vi "Build Application with API.vi"(8 "error in (no error)":errorcluster, 11 "PostBuildSupport in":refnum<class "PostBuildSupport.lvclass">) -> (0 "error out":errorcluster, 3 "PostBuildSupport out":refnum<class "PostBuildSupport.lvclass">)   [LabVIEW 2016, in "PostBuildSupport.lvclass"]
uses:
  PostBuildSupport.lvclass
  PostBuildSupport.lvclass/PostBuildSupport.ctl
  <vilib>/AppBuilder/AB_API/EXE/NI_AB_API_EXE.lvclass
panel:
  in  "Cancel Button":bool
  out "Progress Bar":u8(slide) caption="The build is complete. You can locate the build at\nC:\\user\\patrick\\git\\PPMS-Monitor-and-Control\\builds\\PPMS Monitor and Control\\Application." scale=0.0..100.0
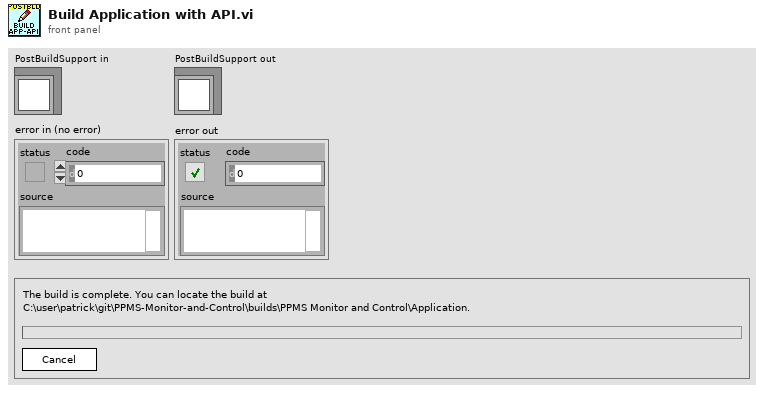
[diagram p1: front panel]
types:
  T1 = enum8{"Enabled", "Disabled", "Disabled and Grayed Out"}
  T2 = typedef "AB_API ProgressBar_Events.ctl" = cluster{"newJob":refnum<user-event>, "newItem":refnum<user-event>, "errorMsg":T3, "cancel":refnum<user-event>}
  T3 = typedef "AB_API ProgressBar_BuildError.ctl" = refnum<user-event>
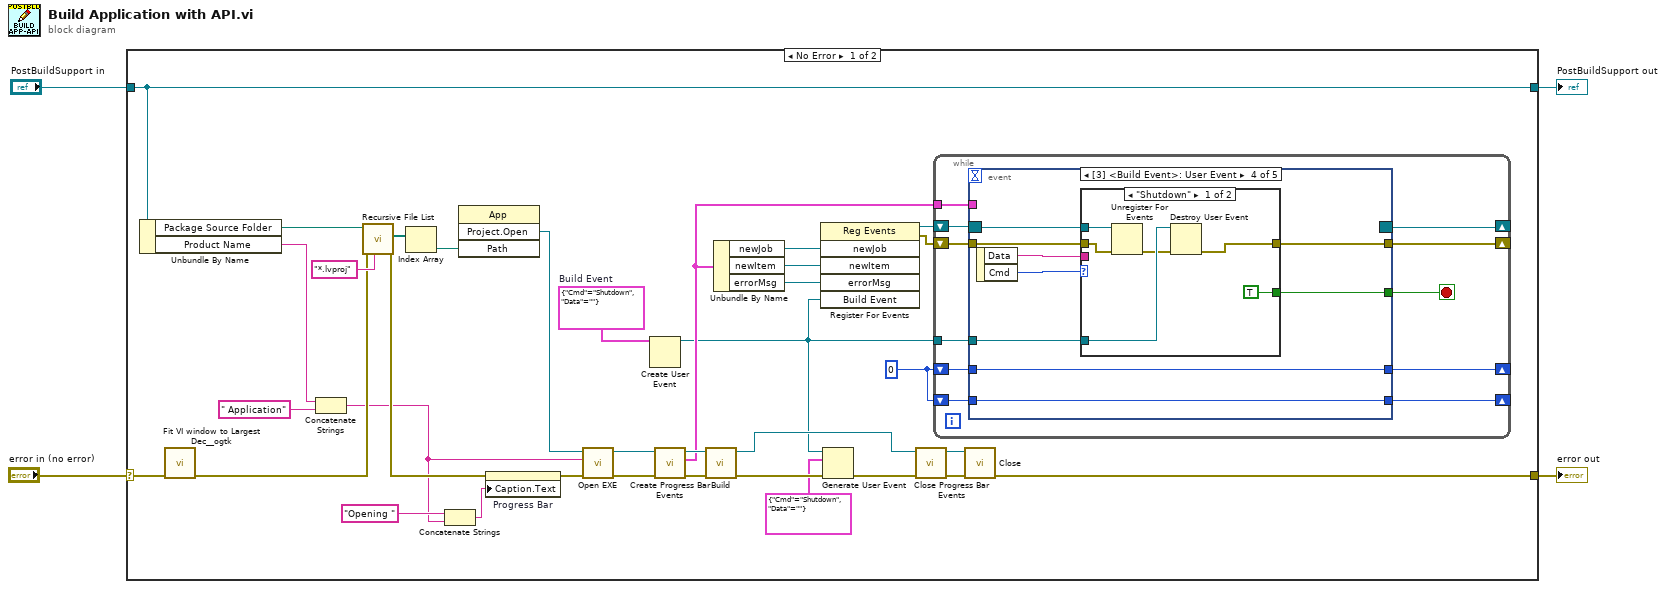
[diagram p0: block diagram]
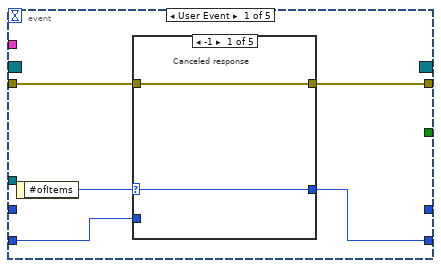
[diagram p2: hidden frame]
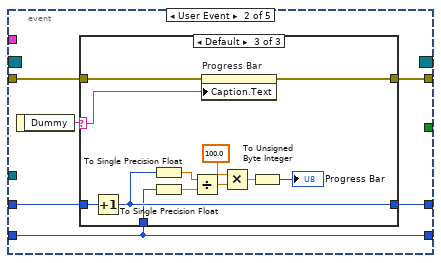
[diagram p7: hidden frame]
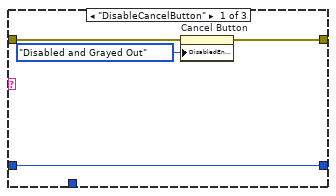
[diagram p8: hidden frame]
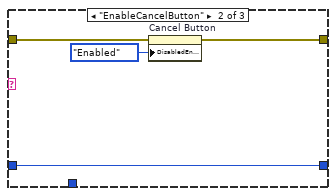
[diagram p9: hidden frame]
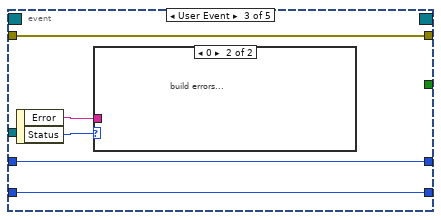
[diagram p10: hidden frame]
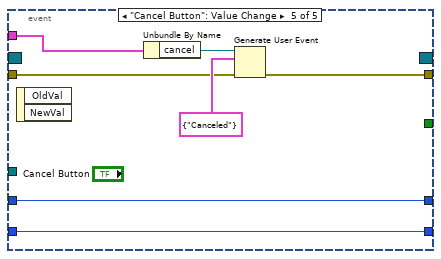
[diagram p13: hidden frame]
diagram:
  n1 = case shown="No Error" "error in (no error)" {
    selector: "error in (no error)" -> [w30 w121]
    tunnel: "PostBuildSupport in" -> [w38 w120]
    tunnel: [w36 w121] -> w2
    tunnel: [w38 w120] -> w1
    frame No Error {
      w19 = cluster{"Cmd":enum16{"Shutdown"}, "Data":string} {"Cmd"=enum."Shutdown", "Data"=""}  # Build Event
      w18 = 0 ("#ofItems")
      n2 = Unbundle By Name(w38) -> ("Package Source Folder"=w32:path, "Product Name"=w33:string)
      n3 = call <userlib>:"Fit VI window to Largest Dec__ogtk.vi"("error in (no error)"=w30) -> ("error out"=w7:errorcluster)  [unwired: 5 in, 1 out]
      n4 = Concatenate Strings(w33, " Application" ("Name of target (My Computer)")) -> (w5:string)
      n5 = call <vilib>:"Recursive File List.vi"("pattern"="*.lvproj", "error in (no error)"=w7, "Folder Path"=w32) -> ("error out"=w6:errorcluster, "All Files in Dir"=w39:path[])  [unwired: 4 in, 3 out]
      n6 = Index Array(array=w39) -> (element=w35:path)  [unwired: 1 in]
      n7 = Concatenate Strings("Opening " ("string"), w5) -> (w9:string)
      n8 = invoke class="App" method="Project.Open"("Path"=w35) -> ("Project:Open"=w34:refnum<vi>)  [unwired: 3 in, 3 out]
      n9 = property on="Progress Bar" class="Slide (strict)"(error in=w6, "Caption.Text"=w9) -> (error out=w10:errorcluster)  [unwired: 1 in, 1 out]
      n10 = call <vilib>:"Open EXE.vi"("error in (no error)"=w10, "Build specification name"=w5, "Project Refnum"=w34) -> ("error out"=w11:errorcluster, "EXE out"=w12:refnum<class "NI_AB_API_EXE.lvclass">)  [unwired: 7 in]
      n11 = Create User Event(user event datatype=w19) -> (user event=w14:refnum<user-event>)  [unwired: 1 in, 1 out]
      n12 = call-dynamic "Create Progress Bar Events.vi"("error in (no error)"=w11, "NI_AB_API_Build in"=w12) -> ("error out"=w25:errorcluster, "progressBarEvents"=w17:T2, "NI_AB_API_Build out"=w29:refnum<class "NI_AB_API_EXE.lvclass">)  [unwired: 7 in]
      n13 = call-dynamic "Build.vi"("error in (no error)"=w25, "EXE in"=w29) -> ("error out"=w16:errorcluster, "EXE out"=w28:refnum<class "NI_AB_API_EXE.lvclass">)  [unwired: 6 in, 2 out]
      n14 = Unbundle By Name(w17) -> ("newJob"=w24:refnum<user-event>, "newItem"=w23:refnum<user-event>, "errorMsg"=w22:T3)
      n15 = register-events(w24, w23, w22, w14) -> (reference out=w21:refnum<event-registration>, error out=w20:errorcluster)  [unwired: 2 in]
      n16 = Generate User Event(user event=w14, event data cluster=cluster{"Cmd":enum16{"Shutdown"}, "Data":string} {"Cmd"=enum."Shutdown", "Data"=""} ("event data"), error in=w16) -> (error out=w15:errorcluster)  [unwired: 1 in, 1 out]
      n17 = call-dynamic "Close Progress Bar Events.vi"("error in (no error)"=w15, "NI_AB_API_Build in"=w28) -> ("error out"=w26:errorcluster, "NI_AB_API_Build out"=w27:refnum<class "NI_AB_API_EXE.lvclass">)  [unwired: 8 in]
      n18 = while {
        shift-right: [w50] -> _
        shift-left: w20 -> [w47]
        shift-right: [w49] -> _
        shift-left: w21 -> [w48]
        shift-right: [w45] -> _
        shift-left: w18 -> [w42]
        shift-right: [w44] -> _
        shift-left: w18 -> [w43]
        tunnel: w14 -> [w41]
        tunnel: w17 -> [w40]
        stop <- w46 stop-if-true
        n19 = event shown="[3] <Build Event>: User Event" {
          selector: w48 -> [_ _ _ w101 _]
          dyn-events: [_ _ _ _ _] -> w49
          timeout: _ -> [_ _ _ _ _]
          tunnel: [w54 w67 w96 w100 w117] -> w50
          tunnel: w47 -> [w55 w66 w96 w99 w113]
          tunnel: [_ _ _ w103 _] -> w46
          tunnel: [w52 w69 w94 w104 w116] -> w45
          tunnel: [_ w70 w95 w105 w115] -> w44
          tunnel: w43 -> [_ w68 w95 w105 w115]
          tunnel: w42 -> [w51 w69 w94 w104 w116]
          tunnel: w41 -> [_ _ _ w97 _]
          tunnel: w40 -> [_ _ _ _ w114]
          event User Event {
            n20 = event-data() -> ("#ofItems"=w53:i32)  [unwired: 1 in]
            n21 = case shown="-1" w53 {
              selector: w53 -> [w57 w59 w61 _ w65]
              tunnel: w55 -> [w56 w58 w60 w63 w64]
              tunnel: [w56 w58 w60 w63 w64] -> w54
              tunnel: [w57 w59 w61 w62 w65] -> w52
              tunnel: w51 -> [_ _ _ w62 _]
              frame -1 {
                # "Canceled response"
              }
              frame -2 {
              }
              frame -3 {
              }
              frame -4 {
              }
              frame Default {
              }
            }
          }
          event User Event {
            n22 = event-data() -> ("Dummy"=w71:string)  [unwired: 1 in]
            n23 = case shown="Default" w71 {
              selector: w71 -> [_ _ w82]
              tunnel: w68 -> [w74 w78 w89]
              tunnel: [w74 w78 w88] -> w70
              tunnel: w69 -> [_ _ w87]
              tunnel: [w72 w76 w80] -> w67
              tunnel: w66 -> [w73 w77 w81]
              frame "DisableCancelButton" {
                n24 = property on="Cancel Button" class="Bool"(error in=w73, "DisabledEnum"=T1."Disabled and Grayed Out" ("Disabled")) -> (error out=w72:errorcluster)  [unwired: 1 in, 1 out]
              }
              frame "EnableCancelButton" {
                n25 = property on="Cancel Button" class="Bool"(error in=w77, "DisabledEnum"=T1."Enabled" ("Disabled")) -> (error out=w76:errorcluster)  [unwired: 1 in, 1 out]
              }
              frame Default {
                n26 = Increment(x=w89) -> (x+1=w88:i32)
                n27 = To Single Precision Float(number=w88) -> (single precision float=w85:sgl)
                n28 = To Single Precision Float(number=w87) -> (single precision float=w84:sgl)
                n29 = Divide(x=w85, y=w84) -> (x/y=w86:sgl)
                n30 = property on="Progress Bar" class="Slide (strict)"(error in=w81, "Caption.Text"=w82) -> (error out=w80:errorcluster)  [unwired: 1 in, 1 out]
                n31 = Multiply(x=sgl 100.0, y=w86) -> (x*y=w91:sgl)
                n32 = To Unsigned Byte Integer(number=w91) -> (unsigned 8bit integer=→"Progress Bar":u8)
              }
            }
          }
          event User Event {
            n33 = event-data() -> ("Error"=w92:string, "Status"=w93:i32)  [unwired: 1 in]
            n34 = case shown="0" w93 {
              tunnel: w92 -> [_ _]
              frame Default {
              }
              frame 0 {
                # "build errors..."
              }
            }
          }
          event User Event {
            n35 = event-data() -> ("Data"=w98:string, "Cmd"=w102:enum16{"Shutdown"})  [unwired: 1 in]
            n36 = case shown="\"Shutdown\"" w102 {
              tunnel: [TRUE _] -> w103
              tunnel: w101 -> [w110 _]
              tunnel: [w106 w112] -> w100
              tunnel: w99 -> [w109 w112]
              tunnel: w98 -> [_ _]
              tunnel: w97 -> [w108 _]
              frame "Shutdown" {
                n37 = Unregister For Events(event registration refnum=w110, error in=w109) -> (error out=w107:errorcluster)
                n38 = Destroy User Event(user event=w108, error in=w107) -> (error out=w106:errorcluster)
              }
              frame Default {
              }
            }
          }
          event "Cancel Button": Value Change {
            n39 = event-data() -> ()  [unwired: 1 in, 2 out]
            n40 = Unbundle By Name(w114) -> ("cancel"=w118:refnum<user-event>)
            n41 = Generate User Event(user event=w118, event data cluster=cluster{"Dummy":string} {"Dummy"="Canceled"} ("event data"), error in=w113) -> (error out=w117:errorcluster)  [unwired: 1 in, 1 out]
          }
        }
      }
      n42 = call-dynamic "Close.vi"("error in (no error)"=w26, "EXE in"=w27) -> ("error out"=w36:errorcluster)  [unwired: 9 in]
    }
    frame Error {
    }
  }
  "error out" <- w2
  "PostBuildSupport out" <- w1
